vi "CodigoLabView 4.vi"() -> (11 "Releb 2":bool)   [LabVIEW 2025]
uses:
  <vilib>/Utility/NIReport.llb/Report Type.ctl
  <vilib>/Instr/_visa.llb/VISA Configure Serial Port (Instr).vi
  <vilib>/addons/_office/excel.llb/Excel Easy Table (str).vi
  <vilib>/Utility/NIReport.llb/NI_report.lvclass
  <vilib>/addons/_office/NI_ReportGenerationToolkit.lvlib
  <vilib>/Utility/NIReport.llb/NI_ReportGenerationCore.lvlib
  <vilib>/Utility/NIReport.llb/Excel/NI_Excel.lvclass
panel:
  out "RI 4":bool
  out "RI 3":bool
  out "RI 2":bool
  out "RS 4":bool
  out "RS 3":bool
  out "RS 2":bool
  out "RS 1":bool
  out "RI 1":bool
  out "errorout":errorcluster
  out "Vrno":refnum<visa-resource-name>
  out "Texto":path=path "C:/Users/Lucas Navarro/Desktop/Ruka/ME2/pf/Jamon.txt"
  out "Historial Tensión de Línea":dbl[](graph)
  out "Historial Tomacorriente 4":dbl[](graph)
  out "Historial Tomacorriente 3":dbl[](graph)
  out "Historial Tomacorriente 2":dbl[](graph)
  out "Historial Tomacorriente 1":dbl[](graph)
  in  "?":bool
  in  "RUTA DE REGISTRO":path
  out "NP4":dbl(knob) scale=0.0..100.0
  out "NP3":dbl(knob) scale=0.0..100.0
  out "NP2":dbl(knob) scale=0.0..100.0
  out "R ON 4":bool
  out "R ON 3":bool
  out "R ON 2":bool
  out "ST":string
  out "R ON 1":bool
  out "NT":dbl(knob) scale=100.0..300.0
  out "NP1":dbl(knob) scale=0.0..100.0
  out "Releb 4":bool
  out "Relea 4":bool
  out "Rele 4":bool
  out "T4":bool
  out "Estado 4":string
  in  "Relé N°4":bool
  out "SP4":string
  out "Releb 3":bool
  out "Relea 3":bool
  out "Rele 3":bool
  out "T3":bool
  out "Estado 3":string
  out "SP3":string
  in  "Relé N°3":bool
  out "Relea 2":bool
  out "Rele 2":bool
  out "T2":bool
  out "Estado 2":string
  out "SP2":string
  in  "Relé N°2":bool
  out "Releb 1":bool
  out "Relea 1":bool
  out "Rele 1":bool
  out "T1":bool
  out "Estado 1":string
  out "SP1":string
  in  "Relé N°1":bool
  in  "PUERTO DE COMUNICACIÓN":refnum<visa-resource-name>
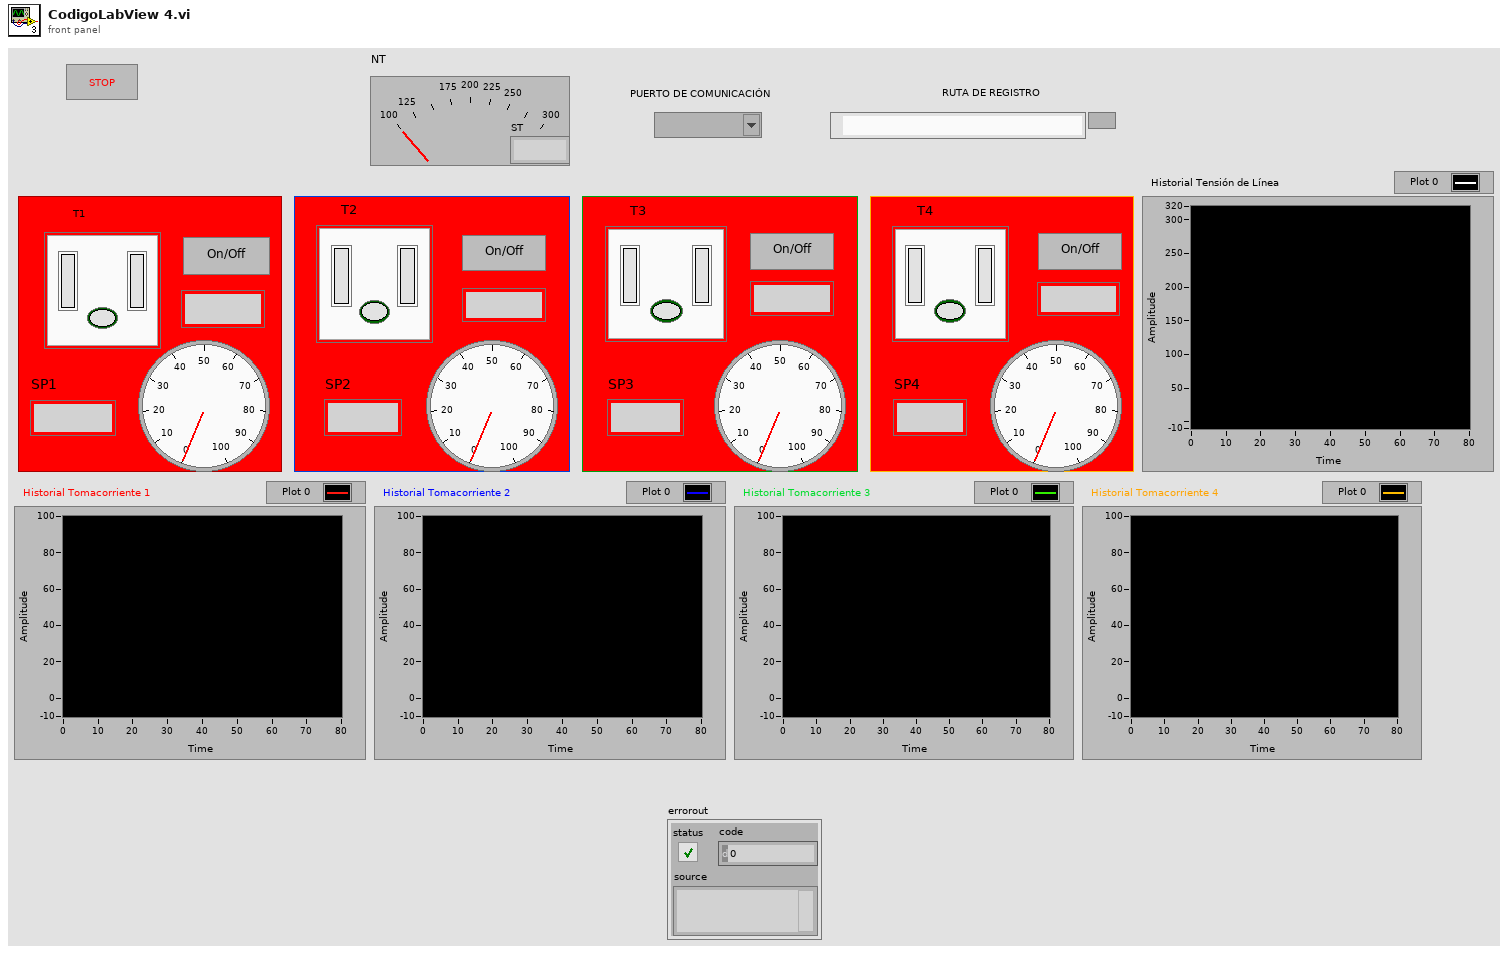
[diagram p1: front panel]
types:
  T1 = typedef "NI_ReportGenerationCore.lvlib/Report Type.ctl" = enum16{"HTML", "Word", "Excel"}
  T2 = cluster{"W1":string, "W2":string, "W3":string, "W4":string, "V":string}
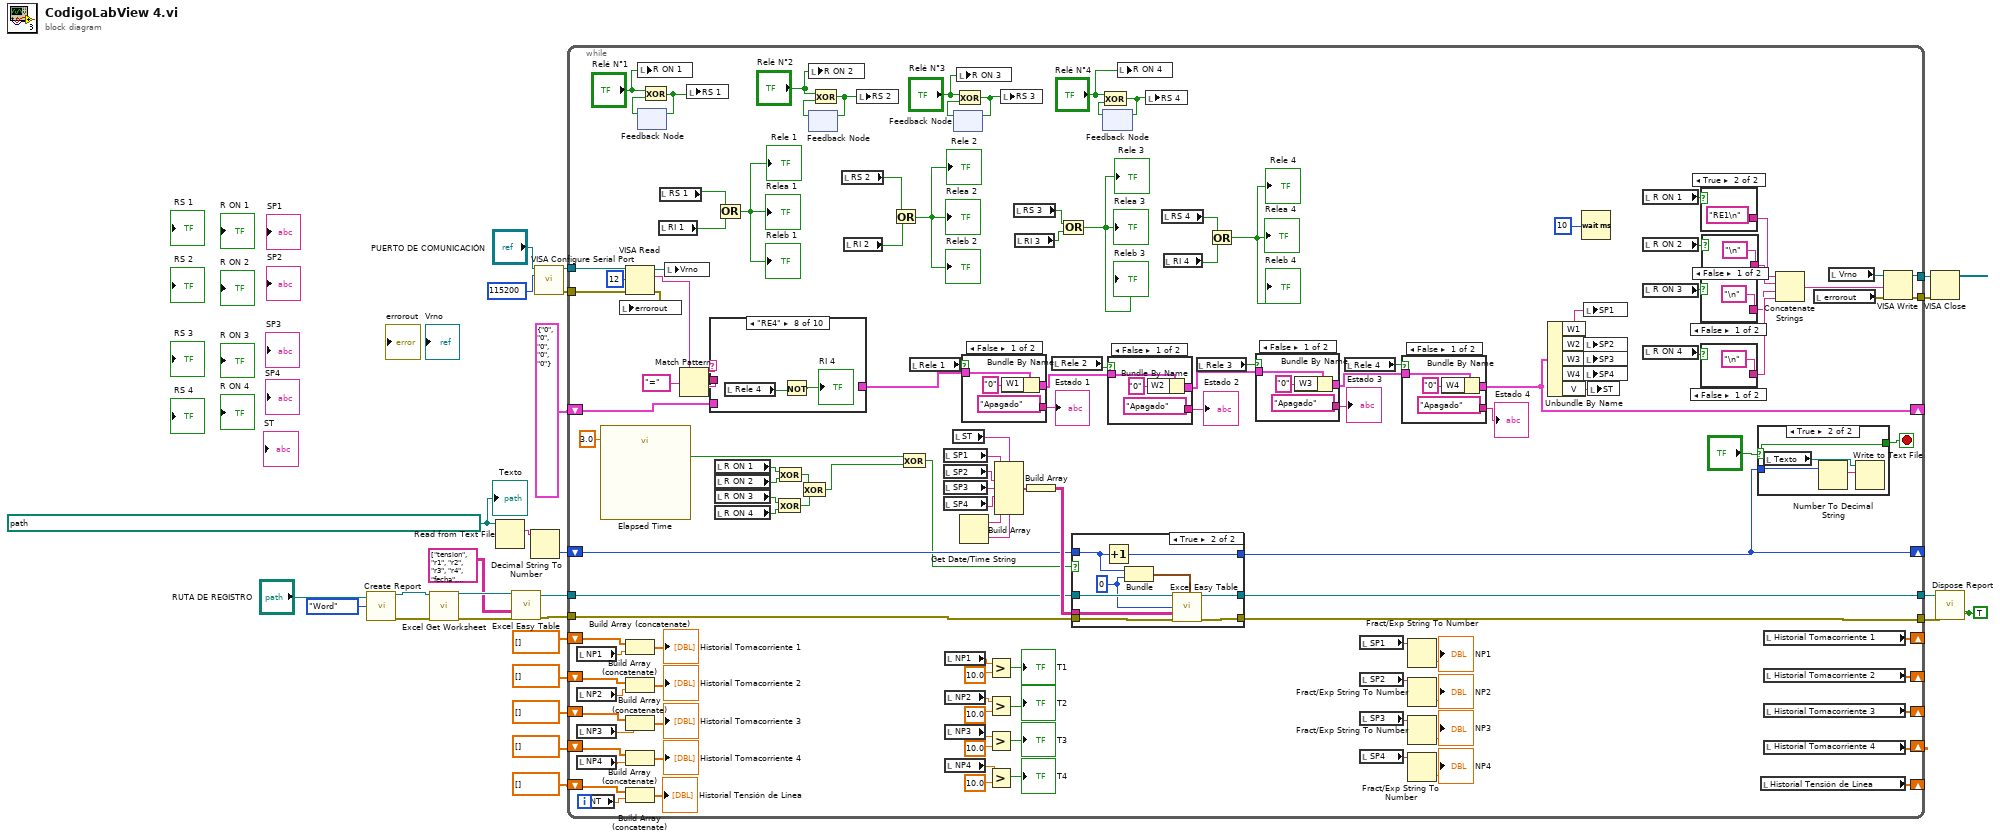
[diagram p0: block diagram]
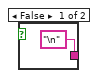
[diagram p2: hidden frame]
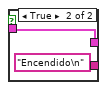
[diagram p3: hidden frame]
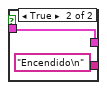
[diagram p4: hidden frame]
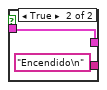
[diagram p5: hidden frame]
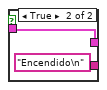
[diagram p8: hidden frame]
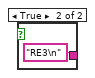
[diagram p9: hidden frame]
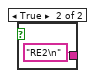
[diagram p10: hidden frame]
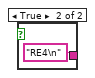
[diagram p11: hidden frame]
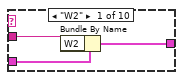
[diagram p12: hidden frame]
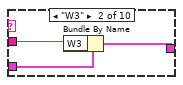
[diagram p13: hidden frame]
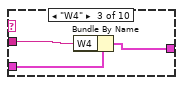
[diagram p14: hidden frame]
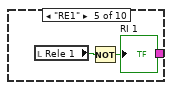
[diagram p16: hidden frame]
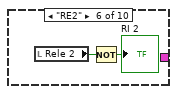
[diagram p17: hidden frame]
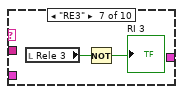
[diagram p18: hidden frame]
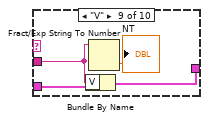
[diagram p19: hidden frame]
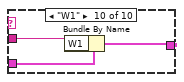
[diagram p20: hidden frame]
diagram:
  w2 = path "C:/Users/drati/Desktop/Santi/Facultad/Medidas Electrónicas II/Proyecto/LabView/registro.txt" ("file (use dialog)")
  w1 = TRUE ("close report? (T)")
  n1 = call <vilib>:"Create Report.vi"("report type"=Report_Type."Word", "template (empty)"="RUTA DE REGISTRO") -> ("report out"=w18:refnum<class "NI_report.lvclass">, "error out"=w17:errorcluster)  [unwired: 12 in]
  n2 = call <vilib>:"Excel Get Worksheet.vi"("report in"=w18, "error in (no error)"=w17) -> ("report out"=w16:refnum<class "NI_report.lvclass">, "error out"=w15:errorcluster)  [unwired: 12 in]
  n3 = Read from Text File(file (use dialog)=w2) -> (text=w9:string)  [unwired: 3 in, 3 out]
  n4 = call-poly <vilib>:"Excel Easy Table.vi"("report in"=w16, "text data"=string[][] [["tension", "r1", "r2", "r3", "r4", "fecha", "hora"]], "error in (no error)"=w15) -> ("report out"=w13:refnum<class "NI_report.lvclass">, "error out"=w12:errorcluster)  [unwired: 8 in, 3 out]
  n5 = Decimal String To Number(string=w9) -> (number=w8:i32)  [unwired: 2 in, 1 out]
  n6 = call-poly "VISA Configure Serial Port"("VISA resource name"="PUERTO DE COMUNICACIÓN", "baud rate (9600)"=u32 115200) -> ("VISA resource name out"=w27:refnum<visa-resource-name>, "error out"=w24:errorcluster)  [unwired: 12 in]
  n7 = while {
    tunnel: w27 -> [w139]
    tunnel: w24 -> [w138]
    shift-right: [w87] -> _
    shift-left: T2 {"W1"="0", "W2"="0", "W3"="0", "W4"="0", "V"="0"} -> [w86]
    tunnel: [w141] -> w22
    tunnel: [w140] -> w21
    shift-right: [w96] -> _
    shift-left: w8 -> [w109]
    tunnel: w13 -> [w130]
    tunnel: w12 -> [w129]
    tunnel: [w122] -> w11
    tunnel: [w121] -> w10
    shift-right: [w43] -> _
    shift-left: dbl[] [] ("array") -> [w118]
    shift-right: [w44] -> _
    shift-left: dbl[] [] ("array") -> [w117]
    shift-right: [w45] -> _
    shift-left: dbl[] [] ("array") -> [w116]
    shift-right: [w47] -> _
    shift-left: dbl[] [] ("array") -> [w115]
    shift-right: [w46] -> _
    shift-left: dbl[] [] ("array") -> [w114]
    stop <- w119 stop-if-true
    n8 = local read "NP1"() -> (w69:dbl)
    n9 = local read "NP2"() -> (w68:dbl)
    n10 = local read "NP3"() -> (w67:dbl)
    n11 = local read "NP4"() -> (w66:dbl)
    n12 = local read "NT"() -> (w65:dbl)
    n13 = call "Elapsed Time"("Time Target (s)"=3.0) -> ("Time has Elapsed"=w41:bool)  [unwired: 11 in, 7 out]
    n14 = VISA Read(VISA resource name=w139, byte count=u32 12 ("Bytes at Port"), error in (no error)=w138) -> (VISA resource name out=w91:refnum<visa-resource-name>, read buffer=w85:string, error out=w90:errorcluster)  [unwired: 1 out]
    n15 = local write "errorout"(w90) -> ()
    n16 = Build Array (concatenate)(w118, w69) -> (→"Historial Tomacorriente 1":dbl[])
    n17 = Build Array (concatenate)(w117, w68) -> (→"Historial Tomacorriente 2":dbl[])
    n18 = Build Array (concatenate)(w116, w67) -> (→"Historial Tomacorriente 3":dbl[])
    n19 = Build Array (concatenate)(w115, w66) -> (→"Historial Tomacorriente 4":dbl[])
    n20 = Build Array (concatenate)(w114, w65) -> (→"Historial Tensión de Línea":dbl[])
    n21 = local write "R ON 1"("Relé N°1") -> ()
    n22 = feedback #1() -> (w157:bool)  [unwired: 1 in]
    n23 = Exclusive Or(1:w157, 2:"Relé N°1") -> (0:w95:bool)
    n24 = feedback-in #1(w95) -> ()
    n25 = local read "RI 1"() -> (w38:bool)
    n26 = local read "RS 1"() -> (w39:bool)
    n27 = local write "Vrno"(w91) -> ()
    n28 = Match Pattern(string=w85, regular expression="=") -> (before substring=w158:string, after substring=w143:string)  [unwired: 1 in, 2 out]
    n29 = local write "RS 1"(w95) -> ()
    n30 = case shown="\"RE4\"" w158 {
      tunnel: w143 -> [w209 w212 w215 _ _ _ _ _ w228 w231]
      tunnel: w86 -> [w211 w214 w217 w218 _ _ _ _ w230 w233]
      tunnel: [w210 w213 w216 w218 _ _ _ _ w229 w232] -> w137
      frame "W2" {
        n31 = Bundle By Name(cluster=w211, "W2"=w209) -> (w210:T2)
      }
      frame "W3" {
        n32 = Bundle By Name(cluster=w214, "W3"=w212) -> (w213:T2)
      }
      frame "W4" {
        n33 = Bundle By Name(cluster=w217, "W4"=w215) -> (w216:T2)
      }
      frame "False", Default {
      }
      frame "RE1" {
        n34 = local read "Rele 1"() -> (w219:bool)
        n35 = Not(x=w219) -> (.not. x?=→"RI 1":bool)
      }
      frame "RE2" {
        n36 = local read "Rele 2"() -> (w222:bool)
        n37 = Not(x=w222) -> (.not. x?=→"RI 2":bool)
      }
      frame "RE3" {
        n38 = local read "Rele 3"() -> (w223:bool)
        n39 = Not(x=w223) -> (.not. x?=→"RI 3":bool)
      }
      frame "RE4" {
        n40 = local read "Rele 4"() -> (w225:bool)
        n41 = Not(x=w225) -> (.not. x?=→"RI 4":bool)
      }
      frame "V" {
        n42 = Bundle By Name(cluster=w230, "V"=w228) -> (w229:T2)
        n43 = Fract/Exp String To Number(string=w228) -> (number=→"NT":dbl)  [unwired: 3 in, 1 out]
      }
      frame "W1" {
        n44 = Bundle By Name(cluster=w233, "W1"=w231) -> (w232:T2)
      }
    }
    n45 = local read "R ON 1"() -> (w128:bool)
    n46 = local read "R ON 2"() -> (w127:bool)
    n47 = local read "R ON 3"() -> (w125:bool)
    n48 = local read "R ON 4"() -> (w126:bool)
    n49 = Or(x=w39, y=w38) -> (x .or. y?=→"Releb 1" →"Relea 1" →"Rele 1":bool)
    n50 = Exclusive Or(1:w126, 2:w125) -> (0:w124:bool)
    n51 = Exclusive Or(1:w127, 2:w128) -> (0:w123:bool)
    n52 = Exclusive Or(1:w124, 2:w123) -> (0:w40:bool)
    n53 = local write "R ON 2"("Relé N°2") -> ()
    n54 = feedback #2() -> (w151:bool)  [unwired: 1 in]
    n55 = Exclusive Or(1:w151, 2:"Relé N°2") -> (0:w94:bool)
    n56 = feedback-in #2(w94) -> ()
    n57 = local read "RS 2"() -> (w36:bool)
    n58 = local read "RI 2"() -> (w35:bool)
    n59 = local write "RS 2"(w94) -> ()
    n60 = Or(x=w36, y=w35) -> (x .or. y?=→"Releb 2" →"Relea 2" →"Rele 2":bool)
    n61 = Exclusive Or(1:w40, 2:w41) -> (0:w42:bool)
    n62 = local read "Rele 1"() -> (w136:bool)
    n63 = local read "SP1"() -> (w73:string)
    n64 = local read "SP2"() -> (w72:string)
    n65 = local read "SP3"() -> (w71:string)
    n66 = local read "SP4"() -> (w70:string)
    n67 = local read "NP1"() -> (w64:dbl)
    n68 = local read "NP2"() -> (w63:dbl)
    n69 = local read "NP3"() -> (w62:dbl)
    n70 = local read "NP4"() -> (w61:dbl)
    n71 = local read "ST"() -> (w74:string)
    n72 = feedback #3() -> (w149:bool)  [unwired: 1 in]
    n73 = Exclusive Or(1:w149, 2:"Relé N°3") -> (0:w93:bool)
    n74 = feedback-in #3(w93) -> ()
    n75 = local write "R ON 3"("Relé N°3") -> ()
    n76 = Get Date/Time String() -> (date string=w134:string, time string=w135:string)  [unwired: 3 in]
    n77 = case shown="False" w136 {
      tunnel: w137 -> [w199 w202]
      tunnel: [w198 w202] -> w107
      tunnel: ["Apagado" "Encendido\n"] -> w100
      frame False {
        n78 = Bundle By Name(cluster=w199, "W1"="0") -> (w198:T2)
      }
      frame True {
      }
    }
    "Estado 1" <- w100
    n79 = Greater?(x=w64, y=10.0) -> (0:→"T1":bool)
    n80 = Greater?(x=w63, y=10.0) -> (0:→"T2":bool)
    n81 = Greater?(x=w62, y=10.0) -> (0:→"T3":bool)
    n82 = Greater?(x=w61, y=10.0) -> (0:→"T4":bool)
    n83 = Build Array(w74, w73, w72, w71, w70, w134, w135) -> (w132:string[])
    n84 = local write "RS 3"(w93) -> ()
    n85 = local read "RS 3"() -> (w33:bool)
    n86 = local read "RI 3"() -> (w32:bool)
    n87 = Build Array(w132) -> (w133:string[][])
    n88 = local read "Rele 2"() -> (w104:bool)
    n89 = Or(x=w33, y=w32) -> (x .or. y?=→"Relea 3" →"Releb 3" →"Rele 3":bool)
    n90 = case shown="True" w42 {
      tunnel: w133 -> [_ w196]
      tunnel: w129 -> [w187 w195]
      tunnel: [w186 w194] -> w122
      tunnel: [w187 w193] -> w121
      tunnel: w130 -> [w186 w192]
      tunnel: w109 -> [w185 w191]
      tunnel: [w185 w190] -> w96
      frame False {
      }
      frame True {
        w188 = 0 ("iteration")
        n91 = Increment(x=w191) -> (x+1=w190:i32)
        n92 = Bundle(w191, "iteration"=w188) -> (w189:cluster{i32, "iteration":i32})  [unwired: 1 in]
        n93 = call-poly <vilib>:"Excel Easy Table.vi"("report in"=w192, "iteration"=w188, "start (0, 0)"=w189, "text data"=w196, "error in (no error)"=w195) -> ("report out"=w194:refnum<class "NI_report.lvclass">, "error out"=w193:errorcluster)  [unwired: 6 in, 3 out]
      }
    }
    n94 = feedback #4() -> (w147:bool)  [unwired: 1 in]
    n95 = Exclusive Or(1:w147, 2:"Relé N°4") -> (0:w92:bool)
    n96 = feedback-in #4(w92) -> ()
    n97 = case shown="False" w104 {
      tunnel: w107 -> [w177 w180]
      tunnel: [w176 w180] -> w106
      tunnel: ["Apagado" "Encendido\n"] -> w98
      frame False {
        n98 = Bundle By Name(cluster=w177, "W2"="0") -> (w176:T2)
      }
      frame True {
      }
    }
    "Estado 2" <- w98
    n99 = local write "R ON 4"("Relé N°4") -> ()
    n100 = local write "RS 4"(w92) -> ()
    n101 = local read "RS 4"() -> (w29:bool)
    n102 = local read "RI 4"() -> (w30:bool)
    n103 = local read "Rele 3"() -> (w103:bool)
    n104 = Or(x=w29, y=w30) -> (x .or. y?=→"Relea 4" →"Releb 4" →"Rele 4":bool)
    n105 = case shown="False" w103 {
      tunnel: w106 -> [w171 w174]
      tunnel: [w170 w174] -> w105
      tunnel: ["Apagado" "Encendido\n"] -> w99
      frame False {
        n106 = Bundle By Name(cluster=w171, "W3"="0") -> (w170:T2)
      }
      frame True {
      }
    }
    "Estado 3" <- w99
    n107 = local read "Rele 4"() -> (w102:bool)
    n108 = local read "SP1"() -> (w78:string)
    n109 = local read "SP2"() -> (w76:string)
    n110 = local read "SP3"() -> (w75:string)
    n111 = local read "SP4"() -> (w77:string)
    n112 = case shown="False" w102 {
      tunnel: w105 -> [w165 w168]
      tunnel: [w164 w168] -> w87
      tunnel: ["Apagado" "Encendido\n"] -> w101
      frame False {
        n113 = Bundle By Name(cluster=w165, "W4"="0") -> (w164:T2)
      }
      frame True {
      }
    }
    "Estado 4" <- w101
    n114 = Fract/Exp String To Number(string=w78) -> (number=→"NP1":dbl)  [unwired: 3 in, 1 out]
    n115 = Fract/Exp String To Number(string=w76) -> (number=→"NP2":dbl)  [unwired: 3 in, 1 out]
    n116 = Fract/Exp String To Number(string=w75) -> (number=→"NP3":dbl)  [unwired: 3 in, 1 out]
    n117 = Fract/Exp String To Number(string=w77) -> (number=→"NP4":dbl)  [unwired: 3 in, 1 out]
    n118 = Unbundle By Name(w87) -> ("W1"=w113:string, "W2"=w110:string, "W3"=w111:string, "W4"=w112:string, "V"=w108:string)
    n119 = Wait (ms)(milliseconds to wait=u32 10) -> ()  [unwired: 1 out]
    n120 = local write "SP1"(w113) -> ()
    n121 = local write "SP2"(w110) -> ()
    n122 = local write "SP3"(w111) -> ()
    n123 = local write "SP4"(w112) -> ()
    n124 = local write "ST"(w108) -> ()
    n125 = local read "R ON 1"() -> (w80:bool)
    n126 = local read "R ON 2"() -> (w154:bool)
    n127 = local read "R ON 3"() -> (w153:bool)
    n128 = local read "R ON 4"() -> (w155:bool)
    n129 = case shown="True" w80 {
      tunnel: ["\n" "RE1\n"] -> w79
      frame False {
      }
      frame True {
      }
    }
    n130 = case shown="False" w153 {
      tunnel: ["\n" "RE3\n"] -> w144
      frame False {
      }
      frame True {
      }
    }
    n131 = case shown="False" w155 {
      tunnel: ["\n" "RE4\n"] -> w145
      frame False {
      }
      frame True {
      }
    }
    n132 = case shown="False" w154 {
      tunnel: ["\n" "RE2\n"] -> w146
      frame False {
      }
      frame True {
      }
    }
    n133 = case shown="True" "?" {
      selector: "?" -> [_ w183]
      tunnel: w96 -> [_ w184]
      tunnel: [_ w183] -> w119
      frame False {
      }
      frame True {
        n134 = local read "Texto"() -> (w181:path)
        n135 = Number To Decimal String(number=w184) -> (decimal integer string=w182:string)  [unwired: 1 in]
        n136 = Write to Text File(file (use dialog)=w181, text=w182) -> ()  [unwired: 2 in, 3 out]
      }
    }
    n137 = local read "Historial Tensión de Línea"() -> (w46:dbl[])
    n138 = local read "Historial Tomacorriente 1"() -> (w43:dbl[])
    n139 = local read "Historial Tomacorriente 2"() -> (w44:dbl[])
    n140 = local read "Historial Tomacorriente 3"() -> (w45:dbl[])
    n141 = local read "Historial Tomacorriente 4"() -> (w47:dbl[])
    n142 = Concatenate Strings(w79, w146, w144, w145) -> (w142:string)
    n143 = local read "errorout"() -> (w89:errorcluster)
    n144 = local read "Vrno"() -> (w88:refnum<visa-resource-name>)
    n145 = VISA Write(VISA resource name=w88, write buffer=w142, error in (no error)=w89) -> (VISA resource name out=w141:refnum<visa-resource-name>, error out=w140:errorcluster)  [unwired: 1 out]
  }
  n146 = VISA Close(VISA resource name=w22, error in (no error)=w21) -> ()  [unwired: 1 out]
  n147 = call-dynamic "Dispose Report.vi"("report in"=w11, "save changes? (F)"=w1, "error in (no error)"=w10, "close report? (T)"=w1) -> ()  [unwired: 11 in, 1 out]
  "Texto" <- w2
